vi "Read Communication.lvclass.vi"(8 "error in (no error)":errorcluster, 11 "Receiver in":refnum<class "Receiver.lvclass">) -> (0 "error out":errorcluster, 2 "Communication.lvclass":refnum<class "Communication.lvclass">, 3 "Receiver out":refnum<class "Receiver.lvclass">)   [LabVIEW 2023, in "Receiver.lvclass"]
uses:
  Receiver.lvclass
  Communication/Communication.lvclass
  Receiver.lvclass/Receiver.ctl
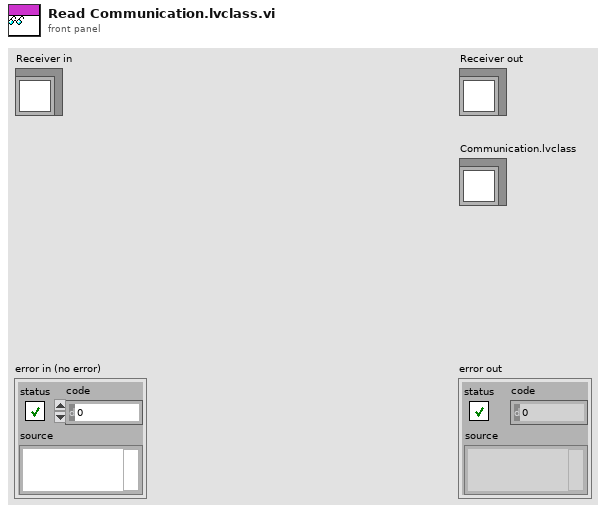
[diagram p1: front panel]
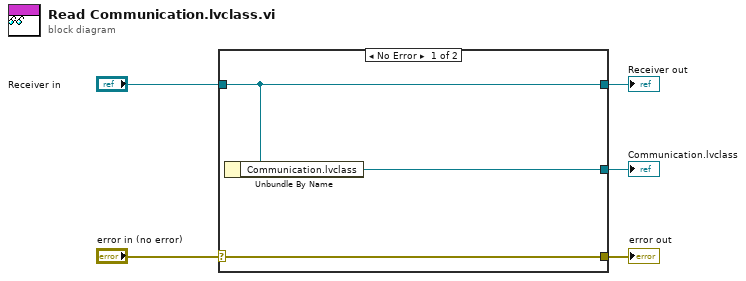
[diagram p0: block diagram]
diagram:
  n1 = case shown="No Error" "error in (no error)" {
    selector: "error in (no error)" -> [w8 w9]
    tunnel: [w8 w9] -> w4
    tunnel: [w7 w10] -> w2
    tunnel: "Receiver in" -> [w7 w10]
    tunnel: [w6 _] -> w1
    frame No Error {
      n2 = Unbundle By Name(w7) -> ("Communication.lvclass"=w6:refnum<class "Communication.lvclass">)
    }
    frame Error {
    }
  }
  "error out" <- w4
  "Receiver out" <- w2
  "Communication.lvclass" <- w1
